vi "sv_Get Window String.vi"(4 "window":T1=1 items=["None"=0, "Hanning"=1, "Hamming"=2, "Blackman-Harris"=3, "Exact Blackman"=4, "Blackman"=5, "Flat Top"=6, "4 Term B-Harris "=7, "7 Term B-Harris"=8, "Low Sidelobe"=9, "Force"=64, "Exponential"=65, "Blackman Nuttall"=11, "Triangle"=30, "Bartlett-Hanning"=31, "Bohman"=32, "Parzen"=33, "Welch"=34, "Kaiser"=60, "Dolph-Chebyshev"=61, "Gaussian"=62]) -> (1 "window string":string)   [LabVIEW 2017]
uses:
  <vilib>/addons/_NISVFA/_Shared subVIs/Controls/svc_Window.ctl
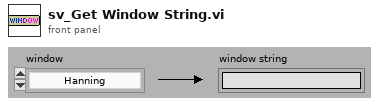
[diagram p1: front panel]
types:
  T1 = typedef "svc_Window.ctl" = u32
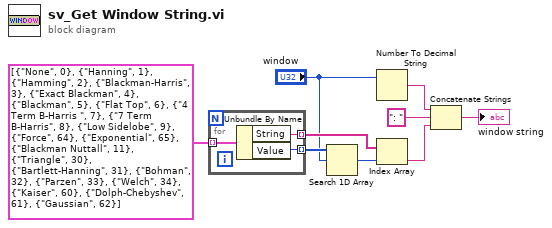
[diagram p0: block diagram]
diagram:
  n1 = for {
    tunnel: cluster{"String":string, "Value":u32}[] [{"String"="None", "Value"=0}, {"String"="Hanning", "Value"=1}, {"String"="Hamming", "Value"=2}, {"String"="Blackman-Harris", "Value"=3}, {"String"="Exact Blackman", "Value"=4}, {"String"="Blackman", "Value"=5}, {"String"="Flat Top", "Value"=6}, {"String"="4 Term B-Harris ", "Value"=7}, {"String"="7 Term B-Harris", "Value"=8}, {"String"="Low Sidelobe", "Value"=9}, {"String"="Force", "Value"=64}, {"String"="Exponential", "Value"=65}, {"String"="Blackman Nuttall", "Value"=11}, {"String"="Triangle", "Value"=30}, {"String"="Bartlett-Hanning", "Value"=31}, {"String"="Bohman", "Value"=32}, {"String"="Parzen", "Value"=33}, {"String"="Welch", "Value"=34}, {"String"="Kaiser", "Value"=60}, {"String"="Dolph-Chebyshev", "Value"=61}, {"String"="Gaussian", "Value"=62}] ("Strings And Values []") -> [w12] mode=indexing
    tunnel: [w11] -> w5 mode=indexing
    tunnel: [w10] -> w4 mode=indexing
    n2 = Unbundle By Name(w12) -> ("String"=w11:string, "Value"=w10:u32)
  }
  n3 = Search 1D Array(1D array=w4, element="window") -> (index of element=w9:i32)  [unwired: 1 in]
  n4 = Number To Decimal String(number="window") -> (decimal integer string=w8:string)  [unwired: 1 in]
  n5 = Index Array(array=w5, index=w9) -> (element=w6:string)
  n6 = Concatenate Strings(w8, ": " ("string"), w6) -> (→"window string":string)
